vi "BusB_Close Hardware References.vi"(8 "error in (no error)":errorcluster, 10 "HW Refnum in":string, 11 "BusB VISA resource":refnum<visa-resource-name>) -> (0 "error out":errorcluster, 2 "HW Refnum out":string)   [LabVIEW 2016, in "Impedance Data Acquisition and Decoding.lvlib"]
uses:
  Impedance Data Acquisition and Decoding.lvlib
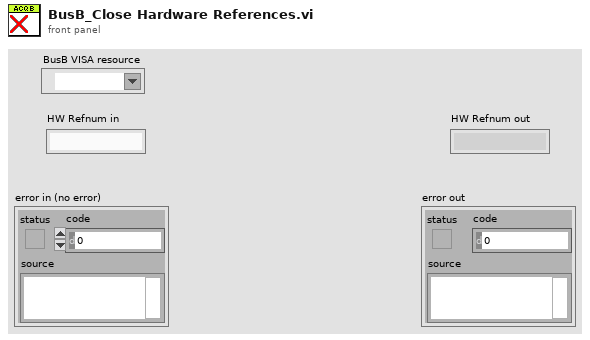
[diagram p1: front panel]
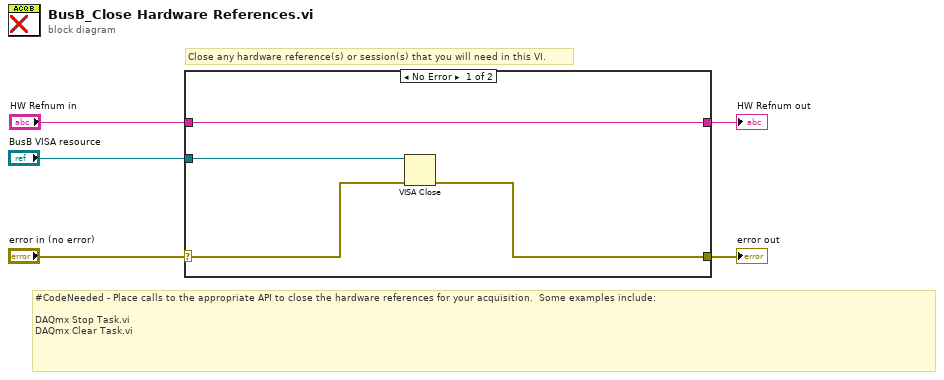
[diagram p0: block diagram]
diagram:
  # "Close any hardware reference(s) or session(s) that you will need in this VI."
  # "#CodeNeeded - Place calls to the appropriate API to close the hardware references for your acquisition.  Some examples include:\n\nDAQmx Stop Task.vi\nDAQmx Clear Task.vi"
  n1 = case shown="No Error" "error in (no error)" {
    selector: "error in (no error)" -> [w8 w10]
    tunnel: [w7 w10] -> w4
    tunnel: "HW Refnum in" -> [w9 w11]
    tunnel: [w9 w11] -> w2
    tunnel: "BusB VISA resource" -> [w6 _]
    frame No Error {
      n2 = VISA Close(VISA resource name=w6, error in (no error)=w8) -> (error out=w7:errorcluster)
    }
    frame Error {
    }
  }
  "HW Refnum out" <- w2
  "error out" <- w4
